vi "PWM RT总.vi"(8 "错误输入（无错误）":errorcluster, 9 "PWM":dbl[](array[numeric])=[1.0, 1.0, 1.0, 1.0], 10 "频率":u16=20000, 11 "Custom FPGA Reference Out":refnum<k20>) -> (0 "错误输出":errorcluster, 3 "FPGA VI引用输出":refnum<k20>)   [LabVIEW 2017]
uses:
  <vilib>/Utility/error.llb/Error Cluster From Error Code.vi
  <vilib>/rvi/errors/niLvFpgaAdjustHostInterfaceError.vi
  <vilib>/rvi/interface/nirviReadWriteControl/nirviReadWriteControl.xnode
  NiFpgaLv.dll
  <vilib>/rvi/interface/Simulation/niFpgaSimulationCallBeginRW.vi
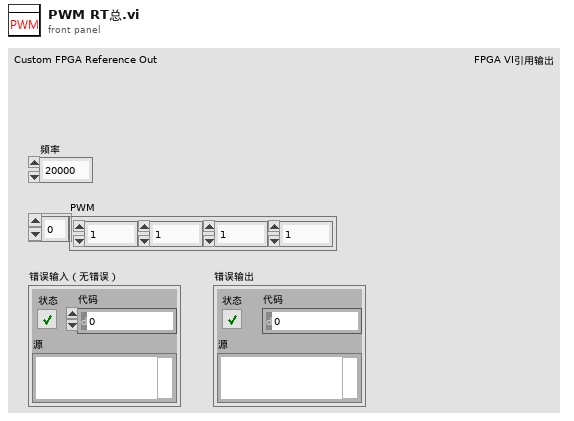
[diagram p1: front panel]
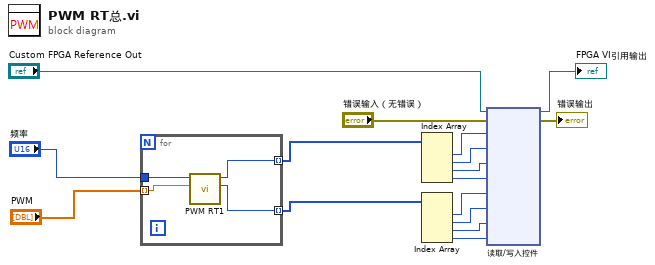
[diagram p0: block diagram]
diagram:
  n1 = for {
    tunnel: "PWM" -> [w20] mode=indexing
    tunnel: [w19] -> w5 mode=indexing
    tunnel: [w18] -> w9 mode=indexing
    tunnel: "频率" -> [w17]
    n2 = call "PWM RT1.vi"("占空比"=w20, "频率"=w17) -> ("F"=w18:u32, "T"=w19:u32)  [unwired: 8 in]
  }
  n3 = Index Array(array=w5) -> (element #1=w6:u32, element #2=w7:u32, element #3=w8:u32, element #4=w3:u32)  [unwired: 4 in]
  n4 = Index Array(array=w9) -> (element #1=w10:u32, element #2=w11:u32, element #3=w12:u32, element #4=w2:u32)  [unwired: 4 in]
  n5 = xnode "读取/写入控件"("FPGA VI引用输入"="Custom FPGA Reference Out", "错误输入"="错误输入（无错误）", "T"=w6, "T 2"=w7, "T 3"=w8, "T 4"=w3, "F"=w10, "F 2"=w11, "F 3"=w12, "F 4"=w2) -> ("FPGA VI引用输出"=→"FPGA VI引用输出":refnum<k20>, "错误输出"=→"错误输出":errorcluster)
